vi "OAT Single Stage Interpolation.vi"(7 "reset? (True)":bool=TRUE, 8 "error in (no error)":errorcluster, 9 "filter":T1={"coefficients"=[], "factor"=1} {"coefficients" format="%.2f"}, 11 "X":dbl[](array[numeric]) format="%.2f") -> (0 "error out":errorcluster, 3 "Y":dbl[](array[numeric]) format="%.2f")   [LabVIEW 2017, in "SoundVib_Resampling.lvlib"]
doc: "Interpolate the input sequence <B>X</B> with the single stage interpolation filter specified by <B>filter</B>."
uses:
  <vilib>/addons/Sound and Vibration/Order Analysis/Resample Order Tracking/SoundVib_Resampling.lvlib
  <vilib>/addons/_NISVFA/_Shared subVIs/Controls/OAT Decimation Filter.ctl
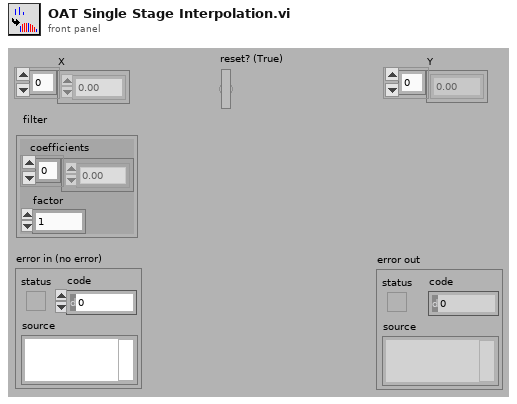
[diagram p1: front panel]
types:
  T1 = typedef "OAT Decimation Filter.ctl" = cluster{"coefficients":dbl[], "factor":i32}
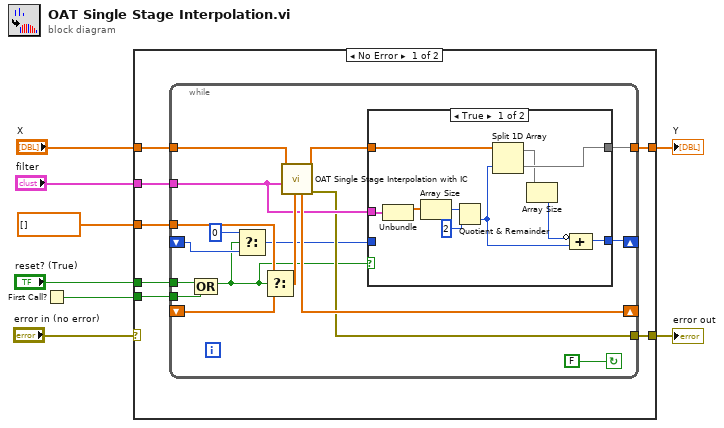
[diagram p0: block diagram]
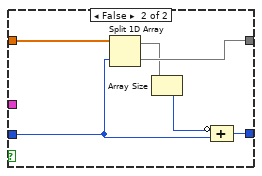
[diagram p2: hidden frame]
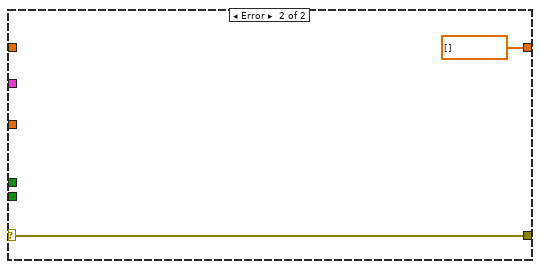
[diagram p3: hidden frame]
diagram:
  n1 = First Call?() -> (First Call?: T/F=w3:bool)
  n2 = case shown="No Error" "error in (no error)" {
    selector: "error in (no error)" -> [_ w50]
    tunnel: "reset? (True)" -> [w15 _]
    tunnel: dbl[] [] ("X[i]") -> [w14 _]
    tunnel: "filter" -> [w13 _]
    tunnel: "X" -> [w12 _]
    tunnel: [w11 dbl[] [] ("Y")] -> w4
    tunnel: w3 -> [w10 _]
    tunnel: [w9 w50] -> w1
    frame No Error {
      n3 = while {
        tunnel: [w26] -> w11
        tunnel: w12 -> [w28]
        tunnel: w13 -> [w22]
        tunnel: w14 -> [w31]
        tunnel: w15 -> [w23]
        shift-left: _ -> [w32]
        shift-right: [w30] -> _
        tunnel: w10 -> [w24]
        tunnel: [w21] -> w9
        shift-right: [w20] -> _
        shift-left: _ -> [w19]
        stop <- FALSE continue-if-true
        n4 = Compound Arithmetic op=OR(w23, w24) -> (w18:bool)
        n5 = Select(t=0, s=w18, f=w19) -> (s? t:f=w16:i32)
        n6 = Select(t=w31, s=w18, f=w32) -> (s? t:f=w29:dbl[])
        n7 = call <vilib>:"OAT Single Stage Interpolation with IC.vi"("initial state"=w29, "filter"=w22, "X"=w28) -> ("error out"=w21:errorcluster, "Y"=w27:dbl[], "final state"=w30:dbl[])  [unwired: 6 in]
        n8 = case shown="True" w18 {
          tunnel: w22 -> [w42 _]
          tunnel: w27 -> [w38 w48]
          tunnel: [w37 w47] -> w26
          tunnel: [w34 w45] -> w20
          tunnel: w16 -> [_ w43]
          frame True {
            n9 = Unbundle(w42) -> ("coefficients"=w41:dbl[])  [unwired: 1 out]
            n10 = Array Size(array=w41) -> (size(s)=w40:i32)
            n11 = Quotient & Remainder(x=w40, y=2) -> (floor(x/y)=w35:i32)  [unwired: 1 out]
            n12 = Split 1D Array(array=w38, index=w35) -> (first subarray=w33:dbl[], second subarray=w37:dbl[])
            n13 = Array Size(array=w33) -> (size(s)=w36:i32)
            n14 = Compound Arithmetic op=ADD(invert w36, w35) -> (w34:i32)
          }
          frame False {
            n15 = Split 1D Array(array=w48, index=w43) -> (first subarray=w44:dbl[], second subarray=w47:dbl[])
            n16 = Array Size(array=w44) -> (size(s)=w46:i32)
            n17 = Compound Arithmetic op=ADD(invert w46, w43) -> (w45:i32)
          }
        }
      }
    }
    frame Error {
    }
  }
  "Y" <- w4
  "error out" <- w1
